vi "Send Request (Async).vi"(8 "error in (no error)":errorcluster, 10 "JSON Request String":string, 11 "Server in":refnum<class "JSONRPC Server.lvclass">) -> (0 "error out":errorcluster, 1 "notification?":bool, 2 "id value":string, 3 "Server out":refnum<class "JSONRPC Server.lvclass">)   [LabVIEW 2015, in "JSONRPC Server.lvclass"]
uses:
  JSONRPC Server.lvclass
  Request/Request.lvclass
  JSONRPC Server.lvclass/JSONRPC Server.ctl
  Request/Request.lvclass/Request.ctl
  Request/Read id value.vi
  id/id.lvclass
  JSONable/JSONable.lvclass
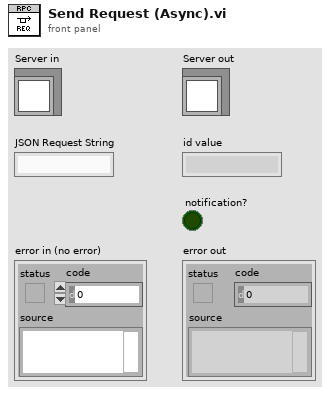
[diagram p1: front panel]
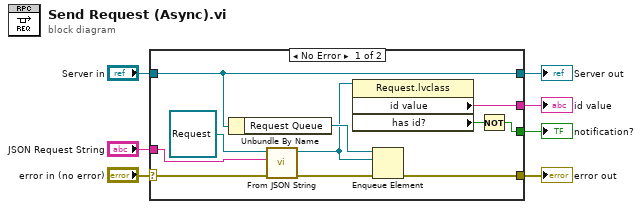
[diagram p0: block diagram]
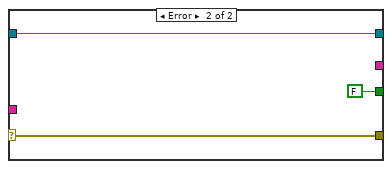
[diagram p2: hidden frame]
diagram:
  n1 = case shown="No Error" "error in (no error)" {
    selector: "error in (no error)" -> [w14 w21]
    tunnel: [w12 w21] -> w6
    tunnel: [w18 w20] -> w4
    tunnel: "Server in" -> [w18 w20]
    tunnel: "JSON Request String" -> [w15 _]
    tunnel: [w10 _] -> w2
    tunnel: [w8 FALSE] -> w1
    frame No Error {
      n2 = Unbundle By Name(w18) -> ("Request Queue"=w17:refnum<queue>)
      n3 = call "From JSON String.vi"("error in (no error)"=w14, "JSON String"=w15, "JSONable in"=refnum<class "Request.lvclass"> refnum ("Request.lvclass")) -> ("error out"=w13:errorcluster, "JSONable out"=w11:refnum<class "Request.lvclass">)  [unwired: 7 in]
      n4 = property class="Request.lvclass"(reference=w11) -> ("id value"=w10:string, "has id?"=w9:bool)  [unwired: 1 in, 2 out]
      n5 = Enqueue Element(queue=w17, element=w11, error in (no error)=w13) -> (error out=w12:errorcluster)  [unwired: 1 in, 2 out]
      n6 = Not(x=w9) -> (.not. x?=w8:bool)
    }
    frame Error {
    }
  }
  "error out" <- w6
  "Server out" <- w4
  "id value" <- w2
  "notification?" <- w1
